vi "Write Alias.vi"(8 "error in (no error)":errorcluster, 10 "Alias":string, 11 "DeployResource in":refnum<class "DeployResource.lvclass">) -> (0 "error out":errorcluster, 3 "DeployResource out":refnum<class "DeployResource.lvclass">)   [LabVIEW 2020, in "PicoG-Core.lvlib" / "DeployResource.lvclass"]
uses:
  DeployResource.lvclass
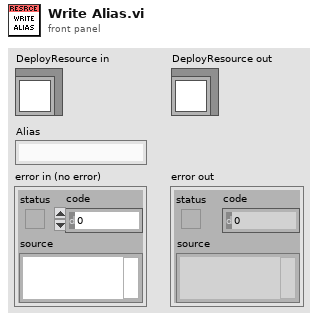
[diagram p1: front panel]
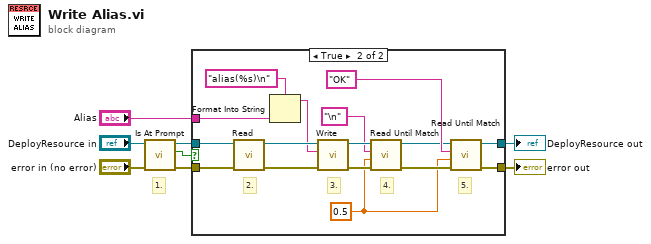
[diagram p0: block diagram]
diagram:
  # "1."
  n1 = call-dynamic "Is At Prompt.vi"("error in (no error)"="error in (no error)", "DeployResource in"="DeployResource in") -> ("error out"=w4:errorcluster, "At Prompt?"=w6:bool, "DeployResource out"=w5:refnum<class "DeployResource.lvclass">)  [unwired: 6 in, 1 out]
  n2 = case shown="True" w6 {
    tunnel: w5 -> [w10 w26]
    tunnel: w4 -> [w9 w25]
    tunnel: [w10 w22] -> w3
    tunnel: [w9 w21] -> w2
    tunnel: "Alias" -> [_ w12]
    frame False {
      # "#ERROR"
    }
    frame True {
      w14 = 0.5 ("Timeout S (0)")
      # "5."
      # "4."
      # "3."
      # "2."
      n3 = call "Read.vi"("error in (no error)"=w25, "DeployResource in"=w26) -> ("error out"=w23:errorcluster, "DeployResource out"=w24:refnum<class "DeployResource.lvclass">)  [unwired: 6 in, 2 out]
      n4 = Format Into String(format string="alias(%s)\n" ("Data"), w12) -> (resulting string=w11:string)  [unwired: 2 in, 1 out]
      n5 = call "Write.vi"("error in (no error)"=w23, "Data"=w11, "DeployResource in"=w24) -> ("error out"=w18:errorcluster, "DeployResource out"=w19:refnum<class "DeployResource.lvclass">)  [unwired: 6 in, 1 out]
      n6 = call "Read Until Match.vi"("error in (no error)"=w18, "Timeout S (0)"=w14, "Match String"="\n" ("Data"), "DeployResource in"=w19) -> ("error out"=w16:errorcluster, "DeployResource out"=w17:refnum<class "DeployResource.lvclass">)  [unwired: 4 in, 2 out]
      n7 = call "Read Until Match.vi"("error in (no error)"=w16, "Timeout S (0)"=w14, "Match String"="OK" ("Data"), "DeployResource in"=w17) -> ("error out"=w21:errorcluster, "DeployResource out"=w22:refnum<class "DeployResource.lvclass">)  [unwired: 4 in, 2 out]
    }
  }
  "error out" <- w2
  "DeployResource out" <- w3
